vi "Read offsetType.vi"(8 "error in (no error)":errorcluster, 11 "OffsetDef in":refnum<class "OffsetDef.lvclass">) -> (0 "error out":errorcluster, 2 "offsetType":T1, 3 "OffsetDef out":refnum<class "OffsetDef.lvclass">)   [LabVIEW 2014, in "TCSDataDefinitions.lvlib" / "TCSCommand.lvlib" / "OffsetCommands.lvlib" / "OffsetDef.lvclass"]
uses:
  OffsetDef.lvclass
  Enumerations/OffsetType.ctl
  OffsetDef.lvclass/OffsetDef.ctl
  OffsetCommands.lvlib
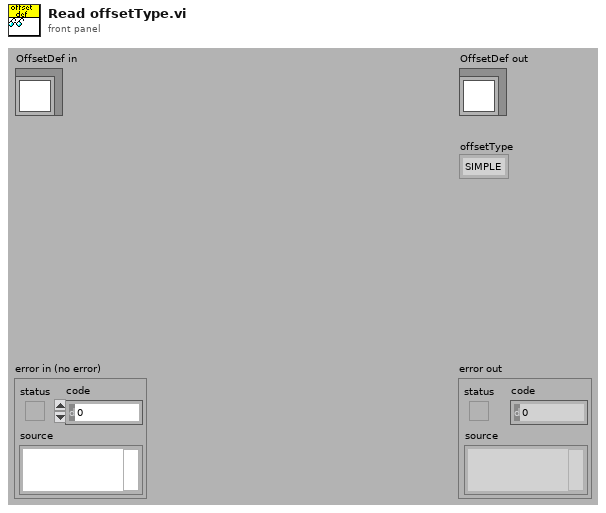
[diagram p1: front panel]
types:
  T1 = typedef "TCSDataDefinitions.lvlib/TCSCommand.lvlib/OffsetCommands.lvlib/OffsetType.ctl" = enum16{"SIMPLE", "TPLANE", "PA"}
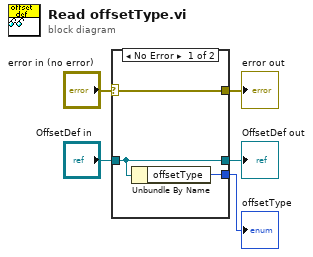
[diagram p0: block diagram]
diagram:
  n1 = case shown="No Error" "error in (no error)" {
    selector: "error in (no error)" -> [w8 w9]
    tunnel: [w8 w9] -> w4
    tunnel: [w7 w10] -> w2
    tunnel: "OffsetDef in" -> [w7 w10]
    tunnel: [w6 _] -> w1
    frame No Error {
      n2 = Unbundle By Name(w7) -> ("offsetType"=w6:T1)
    }
    frame Error {
    }
  }
  "error out" <- w4
  "OffsetDef out" <- w2
  "offsetType" <- w1
